vi "svl_Decimate Resampled Signal (1 Ch).vi"(6 "actual time constant [ms]":dbl format="%.2f", 7 "decimation factor":i32, 8 "error in (no error)":errorcluster, 9 "processing state":T1(ring), 11 "even angle signal":T2 {"even angle signal" format="%.2f"; "dr" format="%.2f"; "r0" format="%.2f"}) -> (0 "error out":errorcluster, 1 "dup actual time constant [ms]":dbl format="%.2f", 3 "even angle signal":T2 {"even angle signal" format="%.2f"; "dr" format="%.2f"; "r0" format="%.2f"}, 5 "actual decimation factor":i32=1 min=1 step=1)   [LabVIEW 2017]
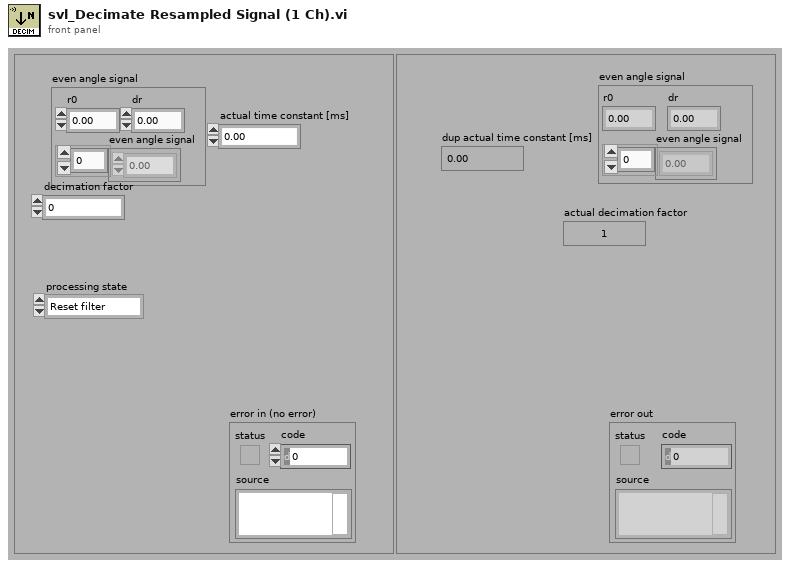
[diagram p1: front panel]
types:
  T1 = enum16{"Reset filter", "Restart averaging", "Continue processing"}
  T2 = cluster{"r0":dbl, "dr":dbl, "even angle signal":dbl[]}
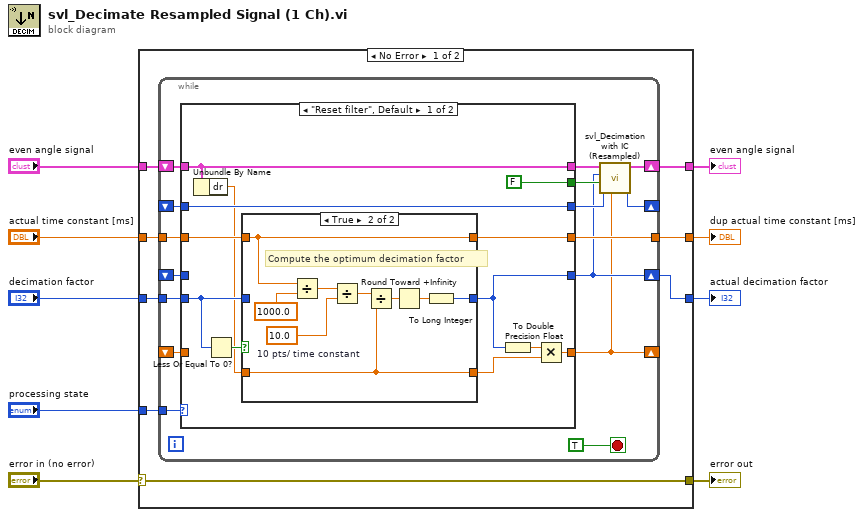
[diagram p0: block diagram]
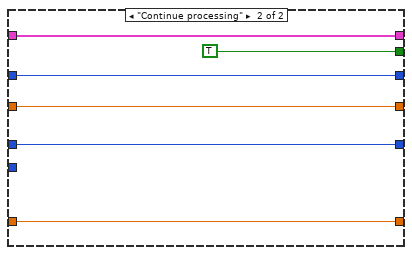
[diagram p3: hidden frame]
diagram:
  n1 = case shown="No Error" "error in (no error)" {
    selector: "error in (no error)" -> [w15 w67]
    tunnel: "decimation factor" -> [w16 w64]
    tunnel: "even angle signal" -> [w14 w66]
    tunnel: [w15 w67] -> w6
    tunnel: [w13 w66] -> w7
    tunnel: [w10 w65] -> w9
    tunnel: "actual time constant [ms]" -> [w12 w65]
    tunnel: "processing state" -> [w17 _]
    tunnel: [w11 w64] -> w1
    frame No Error {
      n2 = while {
        tunnel: [w25] -> w10
        shift-left: _ -> [w27]
        shift-right: [w18] -> _
        shift-left: _ -> [w28]
        shift-right: [w23] -> _
        tunnel: w12 -> [w29]
        shift-left: _ -> [w26]
        shift-right: [w21] -> w11
        tunnel: w16 -> [w31]
        tunnel: w17 -> [w33]
        shift-right: [w19] -> w13
        shift-left: w14 -> [w30]
        stop <- TRUE stop-if-true
        n3 = case shown="\"Reset filter\", Default" w33 {
          tunnel: w31 -> [w44 _]
          tunnel: w30 -> [w34 w60]
          tunnel: [w34 w60] -> w20
          tunnel: w29 -> [w43 w61]
          tunnel: [w36 w59] -> w22
          tunnel: w28 -> [w36 w59]
          tunnel: [w38 w63] -> w18
          tunnel: w27 -> [_ w63]
          tunnel: [w40 w62] -> w21
          tunnel: w26 -> [_ w62]
          tunnel: [w42 w61] -> w25
          tunnel: [FALSE ("init/cont (init:F)") TRUE ("init/cont (init:F)")] -> w24
          frame "Reset filter", Default {
            n4 = Unbundle By Name(w34) -> ("dr"=w35:dbl)
            n5 = Less Or Equal To 0?(x=w44) -> (x <= 0?=w45:bool)
            n6 = case shown="True" w45 {
              tunnel: w44 -> [w47 _]
              tunnel: w35 -> [w46 w49]
              tunnel: [w46 w49] -> w41
              tunnel: [w47 w50] -> w40
              tunnel: w43 -> [w48 w55]
              tunnel: [w48 w55] -> w42
              frame False {
                # "User defined decimation factor"
              }
              frame True {
                w57 = 10.0  # 10 pts/ time constant
                # "Compute the optimum decimation factor"
                n7 = Divide(x=w55, y=1000.0) -> (x/y=w53:dbl)
                n8 = Divide(x=w53, y=w57) -> (x/y=w56:dbl)
                n9 = Divide(x=w56, y=w49) -> (x/y=w52:dbl)
                n10 = Round Toward +Infinity(x=w52) -> (ceil(x): smallest int >= x=w51:dbl)
                n11 = To Long Integer(number=w51) -> (32bit integer=w50:i32)
              }
            }
            n12 = To Double Precision Float(number=w40) -> (double precision float=w39:dbl)
            n13 = Multiply(x=w39, y=w41) -> (x*y=w38:dbl)
          }
          frame "Continue processing" {
          }
        }
        n14 = call <vilib>:"svl_Decimation with IC (Resampled).vi"("new dr"=w18, "initial decimation state"=w22, "init/cont (init:F)"=w24, "decimating factor (1)"=w21, "even angle signal"=w20) -> ("final decimation state"=w23:i32, "even angle signal"=w19:T2)  [unwired: 5 in]
      }
    }
    frame Error {
    }
  }
  "dup actual time constant [ms]" <- w9
  "even angle signal" <- w7
  "error out" <- w6
  "actual decimation factor" <- w1
